vi "MatchRegExSubstringByName.vi"(5 "capture name":string, 7 "Options":cluster{"Compile":u32, "Match":u32} {"Match" format="%.0x"; "Compile" format="%.0x"}, 8 "error in":errorcluster, 9 "offset (0)":u64, 10 "search pattern":string, 11 "string":string) -> (0 "error out":errorcluster, 2 "substring":string, 4 "NextStartOffset":i32, 6 "ContinueMatch?":bool)   [LabVIEW 2021, in "libpcre2-8.lvlib"]
uses:
  libpcre2-8.lvlib
  Pcre2CompileError.vi
  Pcre2ErrorNull.vi
  Pcre2LibError.vi
  Pcre2FnkCallError.vi
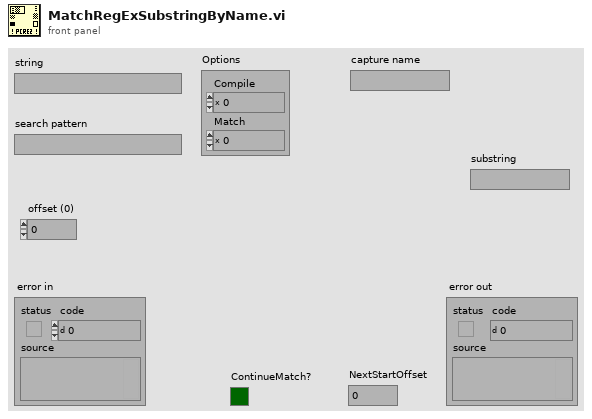
[diagram p1: front panel]
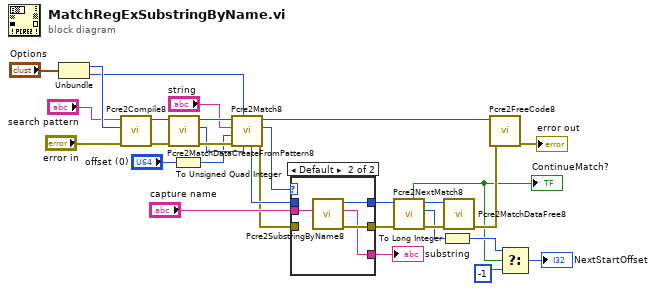
[diagram p0: block diagram]
diagram:
  n1 = Unbundle("Options") -> ("Compile"=w23:u32, "Match"=w22:u32)
  n2 = call "Pcre2Compile8.vi"("error in"="error in", "Options"=w23, "Pattern"="search pattern") -> ("error out"=w28:errorcluster, "pCode"=w27:u64)  [unwired: 7 in]
  n3 = call "Pcre2MatchDataCreateFromPattern8.vi"("error in"=w28, "pCode"=w27) -> ("error out"=w29:errorcluster, "pMatchData"=w21:u64, "pCode"=w30:u64)  [unwired: 7 in]
  n4 = To Unsigned Quad Integer(1:"offset (0)") -> (0:w6:u64)
  n5 = call "Pcre2Match8.vi"("pMatchData"=w21, "Options"=w22, "error in"=w29, "StartOffset"=w6, "Subject"="string", "pCode"=w30) -> ("error out"=w8:errorcluster, "MatchResult"=w10:i32, "pCode"=w2:u64, "pMatchData"=w9:u64)  [unwired: 2 in]
  n6 = case shown="Default" w10 {
    tunnel: w9 -> [w32 _]
    tunnel: [_ w33] -> w15
    tunnel: [w32 w36] -> w14
    tunnel: "capture name" -> [_ w34]
    tunnel: w8 -> [w31 _]
    tunnel: [w31 w35] -> w12
    frame ..-1 {
    }
    frame Default {
      n7 = call "Pcre2SubstringByName8.vi"("Name"=w34) -> ("error out"=w35:errorcluster, "Substring"=w33:string, "pMatchData"=w36:u64)  [unwired: 8 in]
    }
  }
  "substring" <- w15
  n8 = call "Pcre2NextMatch8.vi"("error in"=w12, "pMatchData"=w14) -> ("error out"=w11:errorcluster, "NextStartOffset"=w7:u64, "pMatchData"=w13:u64, "ContinueMatch?"=w1:bool)  [unwired: 5 in, 1 out]
  "ContinueMatch?" <- w1
  n9 = To Long Integer(number=w7) -> (32bit integer=w3:i32)
  n10 = call "Pcre2MatchDataFree8.vi"("error in"=w11, "pMatchData"=w13) -> ("error out"=w26:errorcluster)  [unwired: 9 in]
  n11 = call "Pcre2FreeCode8.vi"("error in"=w26, "pCode"=w2) -> ("error out"=→"error out":errorcluster)  [unwired: 9 in]
  n12 = Select(t=w3, s=w1, f=-1) -> (s? t:f=→"NextStartOffset":i32)
